vi "Apple Gyro Main.vi"(1 "Reset Current":bool, 2 "Reset All":bool, 3 "Override NT?":bool, 4 "Gyro Select (Overide)":enum16{"IMU", "SPI", "Analog", "Navx"}(ring)) -> (0 "Gyro Yaw Out":dbl format="%#_13g")   [LabVIEW 2016, in "Apple Pi Gyro Library.lvlib"]
uses:
  Apple Pi Gyro Library.lvlib
  <vilib>/Rock Robotics/Network Tables/NT Read Number.vi
  <vilib>/Rock Robotics/Network Tables/NT Write Number.vi
  SimpleGyro ADXRS453/SimpleGyro.lvlib
  ADI MXP IMU/ADI MXP IMU/FRC_ADIS16448_IMU.lvlib
  NavX/navX Library v2/navX Library v2.lvlib
panel:
  out "NavX Active":bool
  out "Analog Active":bool
  out "SPI Active":bool
  out "IMU Active":bool
  out "NavX":dbl
  out "Analog":dbl
  out "IMU":dbl
  out "SPI":dbl
  # "Apple Pi 2067 Gyro Library\nBy Chris Garuti\nV 1.0\n\nAllows the selection of 4 different gyrometers through Network Tables"
  # "Active only with Overide on"
  # "All Readings:"
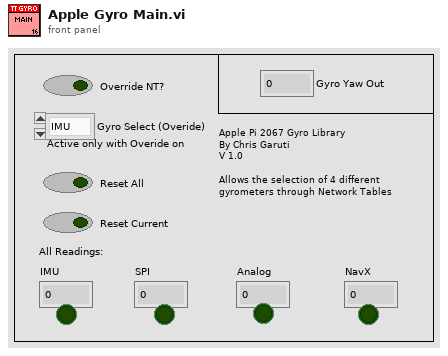
[diagram p1: front panel]
types:
  T1 = typedef "Apple Pi Gyro Library.lvlib/FRC_ADIS16448_IMU.lvlib/WPI_IMU_ADIS16448_InterruptDevRef.ctl" = cluster{"ADI IMU DevRef":T2, "InterruptRef":T4}
  T2 = typedef "Apple Pi Gyro Library.lvlib/FRC_ADIS16448_IMU.lvlib/WPI_IMU_ADIS16448_IMUDevRef.ctl" = cluster{"DevStatus":errorcluster, "Handle":i32, "SPI Bus":T3, "Device Found":bool, "Device Ready":bool, "Yaw Axis":enum16{"X", "Y", "Z"}, "AHRS Algorithm":enum16{"Complementary", "Madgwick"}, "Serial":u16, "Lot ID 2":u16, "Lot ID 1":u16, "Product ID":u16}
  T3 = typedef "spi_bus.ctl" = enum16{"SPI On-Board, CS0", "SPI On-Board, CS1", "SPI On-Board, CS2", "SPI On-Board, CS3", "SPI MXP", "Invalid"}
  T4 = typedef "WPI_InterruptRef.ctl" = cluster{"DevStatus":errorcluster, "InterruptIndex":T5}
  T5 = typedef "FPGA_InterruptIndex.ctl" = enum8{"0", "1", "2", "3", "4", "5", "6", "7", "Invalid"}
  T6 = typedef "Apple Pi Gyro Library.lvlib/SimpleGyro.lvlib/WPI_SimpleGyroDevRef.ctl" = cluster{"DevStatus":errorcluster, "Handle":i32, "SPI Bus":T3, "Device Found":bool, "Sample Rate":dbl}
  T7 = typedef "WPI_GyroDevRef.ctl" = cluster{"DevStatus":errorcluster, "Analog Channel":T8, "Offset":dbl, "Gain (VoltsPerDegree/Second)":dbl, "Gyro Type":enum16{"Analog", "XRS450"}, "Handle":i32, "SPI Bus":T3, "Device Found":bool, "Sample Rate":dbl, "Calibrate On Open":bool}
  T8 = typedef "FPGA_AIChannel.ctl" = enum8{"AI 0", "AI 1", "AI 2", "AI 3", "AI MXP 0", "AI MXP 1", "AI MXP 2", "AI MXP 3", "Invalid"}
  T9 = typedef "Apple Pi Gyro Library.lvlib/navX Library v2.lvlib/Z900_navX_DeviceTypeDef.ctl" = cluster{"Interface":cluster{"Protocol":T10, "Update Rate (4Hz-100Hz)":u8, "navX Open TypeDef":variant}, "Notify Packet":refnum<notifier>, "Loop VI Refnum":refnum<vi>, "Ready to Close Occurrence Refnum":refnum<k4>}
  T10 = typedef "Apple Pi Gyro Library.lvlib/navX Library v2.lvlib/Z900_navX_ProtocolTypeDef.ctl" = enum16{"SERIAL", "I2C", "SPI"}
  T11 = cluster{"Yaw":dbl, "Roll":dbl, "Pitch":dbl, "Heading":dbl, "Fused Heading":dbl}
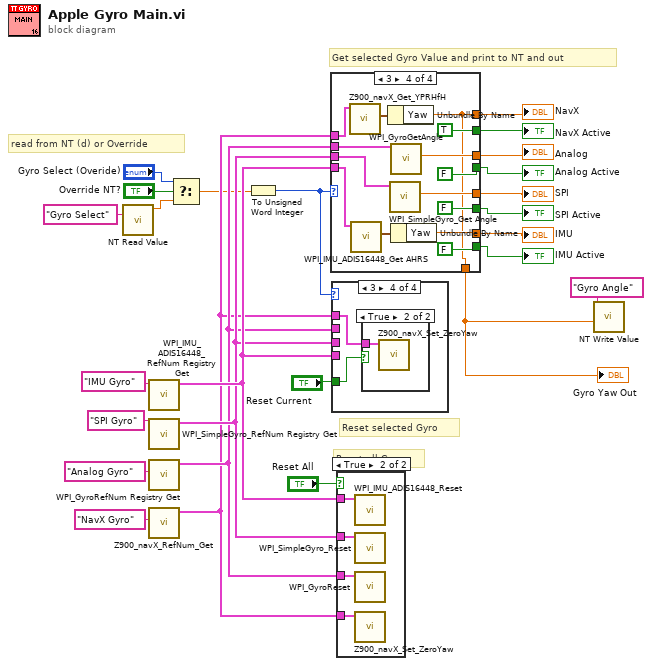
[diagram p0: block diagram]
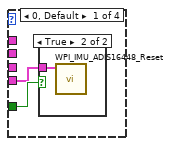
[diagram p3: hidden frame]
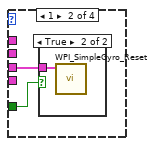
[diagram p5: hidden frame]
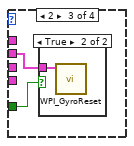
[diagram p7: hidden frame]
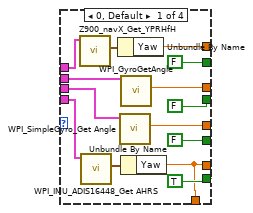
[diagram p10: hidden frame]
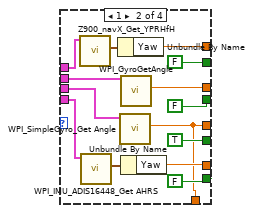
[diagram p11: hidden frame]
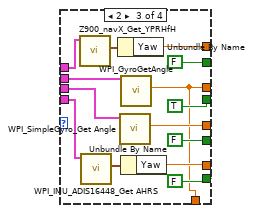
[diagram p12: hidden frame]
diagram:
  # "Get selected Gyro Value and print to NT and out"
  # "read from NT (d) or Override"
  # "Reset all Gyros"
  # "Reset selected Gyro"
  n1 = call-poly <vilib>:"NT Read Value.vi"("Name"="Gyro Select") -> ("Numeric"=w24:dbl)  [unwired: 9 in, 1 out]
  n2 = call "WPI_IMU_ADIS16448_RefNum Registry Get.vi"("refnum name"="IMU Gyro") -> ("ADI IMU Interrupt DevRef"=w18:T1)  [unwired: 9 in, 1 out]
  n3 = call "WPI_SimpleGyro_RefNum Registry Get.vi"("refnum name"="SPI Gyro") -> ("SimpleGyroDevRef"=w17:T6)  [unwired: 9 in, 1 out]
  n4 = call <vilib>:"WPI_GyroRefNum Registry Get.vi"("refnum name"="Analog Gyro") -> ("GyroDevRef"=w13:T7)  [unwired: 9 in, 1 out]
  n5 = call "Z900_navX_RefNum_Get.vi"("refnum name"="NavX Gyro") -> ("navX Device"=w11:T9)  [unwired: 9 in, 1 out]
  n6 = Select(t="Gyro Select (Overide)", s="Override NT?", f=w24) -> (s? t:f=w2:dbl)
  n7 = To Unsigned Word Integer(number=w2) -> (unsigned 16bit integer=w22:u16)
  n8 = case shown="3" w22 {
    tunnel: [w27 w46 w60 w74] -> w7
    tunnel: w18 -> [w39 w53 w67 w81]
    tunnel: w17 -> [w38 w52 w66 w80]
    tunnel: w13 -> [w36 w50 w64 w78]
    tunnel: w11 -> [w35 w49 w63 w77]
    tunnel: [w34 w48 w62 w69] -> w10
    tunnel: [w33 w47 w55 w76] -> w9
    tunnel: [w32 w41 w61 w75] -> w8
    tunnel: [FALSE FALSE FALSE TRUE] -> w6
    tunnel: [FALSE FALSE TRUE FALSE] -> w5
    tunnel: [FALSE TRUE FALSE FALSE] -> w4
    tunnel: [TRUE FALSE FALSE FALSE] -> w3
    tunnel: [w27 w41 w55 w69] -> w1
    frame 0, Default {
      n9 = call "Z900_navX_Get_YPRHfH.vi"("navX Device"=w35) -> ("YRPHfH"=w37:T11)  [unwired: 7 in, 3 out]
      n10 = call "WPI_IMU_ADIS16448_Get AHRS.vi"("ADI IMU Interrupt DevRef"=w39) -> ("IMU AHRS Out"=w40:cluster{"Pitch":dbl, "Roll":dbl, "Yaw":dbl})  [unwired: 6 in, 4 out]
      n11 = Unbundle By Name(w37) -> ("Yaw"=w34:dbl)
      n12 = call "WPI_SimpleGyro_Get Angle.vi"("SimpleGyroDevRef"=w38) -> ("Angle"=w32:dbl)  [unwired: 7 in, 3 out]
      n13 = call <vilib>:"WPI_GyroGetAngle.vi"("GyroDevRef"=w36) -> ("Angle"=w33:dbl)  [unwired: 6 in, 4 out]
      n14 = Unbundle By Name(w40) -> ("Yaw"=w27:dbl)
    }
    frame 1 {
      n15 = call "Z900_navX_Get_YPRHfH.vi"("navX Device"=w49) -> ("YRPHfH"=w51:T11)  [unwired: 7 in, 3 out]
      n16 = call "WPI_IMU_ADIS16448_Get AHRS.vi"("ADI IMU Interrupt DevRef"=w53) -> ("IMU AHRS Out"=w54:cluster{"Pitch":dbl, "Roll":dbl, "Yaw":dbl})  [unwired: 6 in, 4 out]
      n17 = Unbundle By Name(w51) -> ("Yaw"=w48:dbl)
      n18 = call "WPI_SimpleGyro_Get Angle.vi"("SimpleGyroDevRef"=w52) -> ("Angle"=w41:dbl)  [unwired: 7 in, 3 out]
      n19 = call <vilib>:"WPI_GyroGetAngle.vi"("GyroDevRef"=w50) -> ("Angle"=w47:dbl)  [unwired: 6 in, 4 out]
      n20 = Unbundle By Name(w54) -> ("Yaw"=w46:dbl)
    }
    frame 2 {
      n21 = call "Z900_navX_Get_YPRHfH.vi"("navX Device"=w63) -> ("YRPHfH"=w65:T11)  [unwired: 7 in, 3 out]
      n22 = call "WPI_IMU_ADIS16448_Get AHRS.vi"("ADI IMU Interrupt DevRef"=w67) -> ("IMU AHRS Out"=w68:cluster{"Pitch":dbl, "Roll":dbl, "Yaw":dbl})  [unwired: 6 in, 4 out]
      n23 = Unbundle By Name(w65) -> ("Yaw"=w62:dbl)
      n24 = call "WPI_SimpleGyro_Get Angle.vi"("SimpleGyroDevRef"=w66) -> ("Angle"=w61:dbl)  [unwired: 7 in, 3 out]
      n25 = call <vilib>:"WPI_GyroGetAngle.vi"("GyroDevRef"=w64) -> ("Angle"=w55:dbl)  [unwired: 6 in, 4 out]
      n26 = Unbundle By Name(w68) -> ("Yaw"=w60:dbl)
    }
    frame 3 {
      n27 = call "Z900_navX_Get_YPRHfH.vi"("navX Device"=w77) -> ("YRPHfH"=w79:T11)  [unwired: 7 in, 3 out]
      n28 = call "WPI_IMU_ADIS16448_Get AHRS.vi"("ADI IMU Interrupt DevRef"=w81) -> ("IMU AHRS Out"=w82:cluster{"Pitch":dbl, "Roll":dbl, "Yaw":dbl})  [unwired: 6 in, 4 out]
      n29 = Unbundle By Name(w79) -> ("Yaw"=w69:dbl)
      n30 = call "WPI_SimpleGyro_Get Angle.vi"("SimpleGyroDevRef"=w80) -> ("Angle"=w75:dbl)  [unwired: 7 in, 3 out]
      n31 = call <vilib>:"WPI_GyroGetAngle.vi"("GyroDevRef"=w78) -> ("Angle"=w76:dbl)  [unwired: 6 in, 4 out]
      n32 = Unbundle By Name(w82) -> ("Yaw"=w74:dbl)
    }
  }
  "Gyro Yaw Out" <- w1
  "NavX" <- w10
  "NavX Active" <- w6
  "IMU Active" <- w3
  "SPI" <- w8
  "IMU" <- w7
  "Analog Active" <- w5
  "SPI Active" <- w4
  "Analog" <- w9
  n33 = case shown="3" w22 {
    tunnel: "Reset Current" -> [w84 w87 w89 w92]
    tunnel: w18 -> [w83 _ _ _]
    tunnel: w17 -> [_ w86 _ _]
    tunnel: w13 -> [_ _ w90 _]
    tunnel: w11 -> [_ _ _ w93]
    frame 0, Default {
      n34 = case shown="True" w84 {
        tunnel: w83 -> [_ w85]
        frame False {
        }
        frame True {
          n35 = call "WPI_IMU_ADIS16448_Reset.vi"("ADI IMU Interrupt DevRef"=w85) -> ()  [unwired: 9 in, 2 out]
        }
      }
    }
    frame 1 {
      n36 = case shown="True" w87 {
        tunnel: w86 -> [_ w88]
        frame False {
        }
        frame True {
          n37 = call "WPI_SimpleGyro_Reset.vi"("SimpleGyroDevRef"=w88) -> ()  [unwired: 9 in, 2 out]
        }
      }
    }
    frame 2 {
      n38 = case shown="True" w89 {
        tunnel: w90 -> [_ w91]
        frame False {
        }
        frame True {
          n39 = call <vilib>:"WPI_GyroReset.vi"("GyroDevRef"=w91) -> ()  [unwired: 9 in, 2 out]
        }
      }
    }
    frame 3 {
      n40 = case shown="True" w92 {
        tunnel: w93 -> [_ w94]
        frame False {
        }
        frame True {
          n41 = call "Z900_navX_Set_ZeroYaw.vi"("navX Device"=w94) -> ()  [unwired: 9 in, 2 out]
        }
      }
    }
  }
  n42 = case shown="True" "Reset All" {
    tunnel: w18 -> [_ w98]
    tunnel: w17 -> [_ w97]
    tunnel: w13 -> [_ w96]
    tunnel: w11 -> [_ w95]
    frame False {
    }
    frame True {
      n43 = call "WPI_IMU_ADIS16448_Reset.vi"("ADI IMU Interrupt DevRef"=w98) -> ()  [unwired: 9 in, 2 out]
      n44 = call "WPI_SimpleGyro_Reset.vi"("SimpleGyroDevRef"=w97) -> ()  [unwired: 9 in, 2 out]
      n45 = call <vilib>:"WPI_GyroReset.vi"("GyroDevRef"=w96) -> ()  [unwired: 9 in, 2 out]
      n46 = call "Z900_navX_Set_ZeroYaw.vi"("navX Device"=w95) -> ()  [unwired: 9 in, 2 out]
    }
  }
  n47 = call-poly <vilib>:"NT Write Value.vi"("Numeric"=w1, "Name"="Gyro Angle") -> ()  [unwired: 9 in, 1 out]
